vi "Configure Sweep Time.vi"(0 "VISA resource name":refnum<visa-resource-name>, 5 "Sweep Time Mode (0:Normal)":i32(ring) items=["Normal", "Fast"], 7 "Auto Sweep Time (T:Enable)":bool=TRUE, 9 "Sweep Time (100ms)":dbl=100.0 min=0.001 max=999999000.0, 11 "error in (no error)":errorcluster, 12 "Frequency Domain(0:Off)":i32(ring) items=["Off", "On"]) -> (4 "VISA resource name out":refnum<visa-resource-name>, 15 "error out":errorcluster)   [LabVIEW 2020, in "Anritsu Signal Analyzer Series.lvlib"]
doc: "Configures the sweep time settings of the spectrum analyzer."
uses:
  Anritsu Signal Analyzer Series.lvlib
panel:
  # "ms"
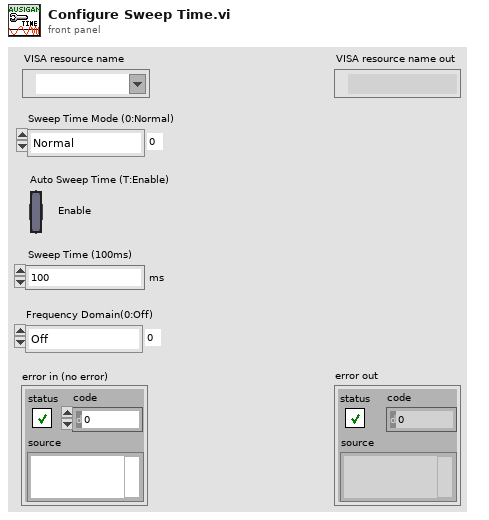
[diagram p1: front panel]
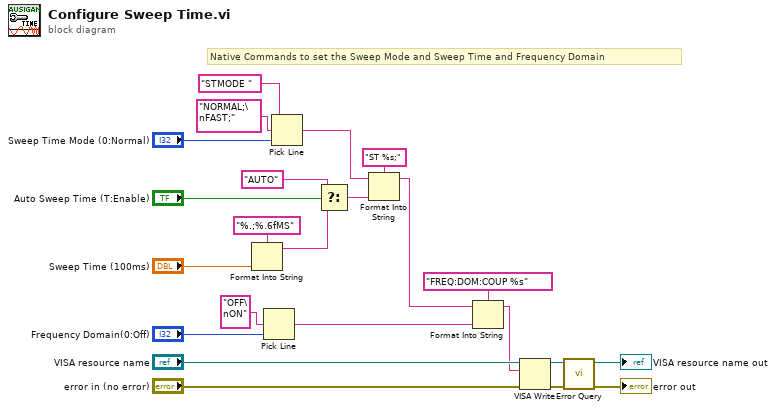
[diagram p0: block diagram]
diagram:
  # "Native Commands to set the Sweep Mode and Sweep Time and Frequency Domain"
  n1 = Format Into String(format string="%.;%.6fMS" ("Format String"), "Sweep Time (100ms)") -> (resulting string=w1:string)  [unwired: 2 in, 1 out]
  n2 = Pick Line(multi-line string="OFF\nON" ("複数行文字列"), line index="Frequency Domain(0:Off)") -> (output string=w9:string)  [unwired: 1 in]
  n3 = Pick Line(string ("")="STMODE " ("_CommandSet"), multi-line string="NORMAL;\nFAST;" ("複数行文字列"), line index="Sweep Time Mode (0:Normal)") -> (output string=w7:string)
  n4 = Select(t="AUTO", s="Auto Sweep Time (T:Enable)", f=w1) -> (s? t:f=w3:string)
  n5 = Format Into String(format string="ST %s;" ("_CommandSet"), initial string=w7, w3) -> (resulting string=w15:string)  [unwired: 1 in, 1 out]
  n6 = Format Into String(format string="FREQ:DOM:COUP %s" ("_CommandSet"), initial string=w15, w9) -> (resulting string=w11:string)  [unwired: 1 in, 1 out]
  n7 = VISA Write(VISA resource name="VISA resource name", write buffer=w11, error in (no error)="error in (no error)") -> (VISA resource name out=w12:refnum<visa-resource-name>, error out=w13:errorcluster)  [unwired: 1 out]
  n8 = call "Error Query.vi"("error in (no error)"=w13, "VISA resource name"=w12) -> ("error out"=→"error out":errorcluster, "VISA resource name out"=→"VISA resource name out":refnum<visa-resource-name>)  [unwired: 6 in, 2 out]
